vi "getCurrentVersion.vi"(8 "error in (no error)":errorcluster, 11 "hgHandler in":refnum<class "hgHandler.lvclass">) -> (0 "error out":errorcluster, 1 "Log":string, 3 "hgHandler out":refnum<class "hgHandler.lvclass">, 4 "Current Version":string)   [LabVIEW 2013, in "hgHandler.lvclass"]
uses:
  hgHandler.lvclass
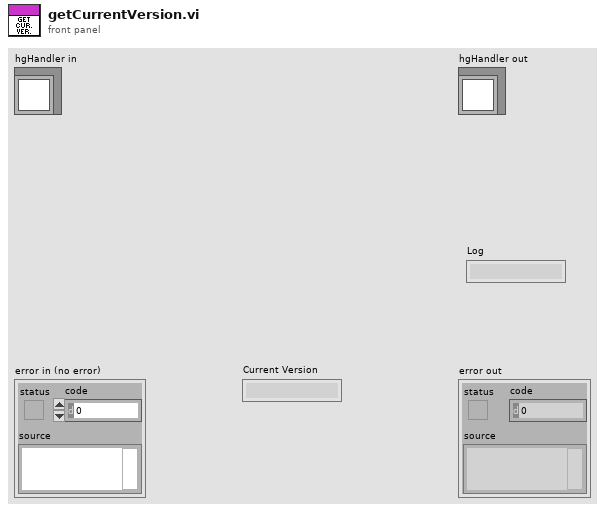
[diagram p1: front panel]
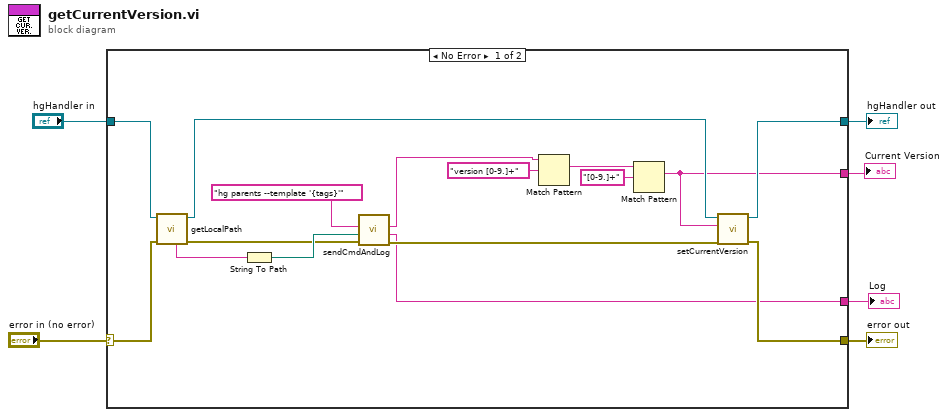
[diagram p0: block diagram]
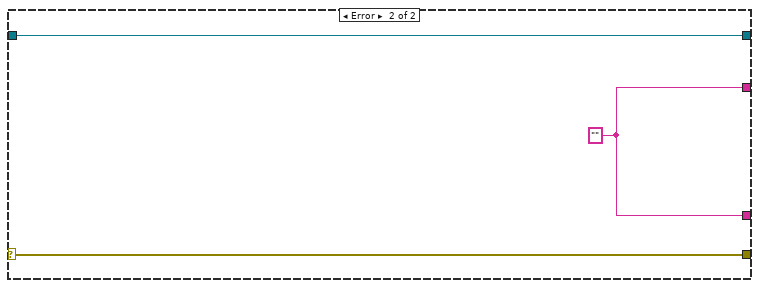
[diagram p2: hidden frame]
diagram:
  n1 = case shown="No Error" "error in (no error)" {
    selector: "error in (no error)" -> [w17 w24]
    tunnel: "hgHandler in" -> [w14 w25]
    tunnel: [w13 w25] -> w4
    tunnel: [w15 w24] -> w3
    tunnel: [w9 w23] -> w2
    tunnel: [w8 w23] -> w1
    frame No Error {
      n2 = call-dynamic "getLocalPath.vi"("error in (no error)"=w17, "repoHandler in"=w14) -> ("error out"=w18:errorcluster, "repoHandler out"=w16:refnum<class "hgHandler.lvclass">, "Local Path"=w7:string)  [unwired: 7 in]
      n3 = String To Path(string=w7) -> (path=w19:path)
      n4 = call "sendCmdAndLog.vi"("error in (no error)"=w18, "working directory"=w19, "command"="hg parents --template '{tags}'" ("command line")) -> ("error out"=w11:errorcluster, "Log"=w9:string, "standard output"=w10:string)  [unwired: 6 in]
      n5 = Match Pattern(string=w10, regular expression="version [0-9.]+") -> (match substring=w20:string)  [unwired: 1 in, 3 out]
      n6 = Match Pattern(string=w20, regular expression="[0-9.]+") -> (match substring=w8:string)  [unwired: 1 in, 3 out]
      n7 = call-dynamic "setCurrentVersion.vi"("error in (no error)"=w11, "Current Version"=w8, "repoHandler in"=w16) -> ("error out"=w15:errorcluster, "repoHandler out"=w13:refnum<class "hgHandler.lvclass">)  [unwired: 7 in]
    }
    frame Error {
      w23 = "" ("Local Version")
    }
  }
  "error out" <- w3
  "hgHandler out" <- w4
  "Current Version" <- w1
  "Log" <- w2
